vi "Simple TCP - Client.vi"() -> ()   [LabVIEW 2017]
doc: "Demonstrates how to open a connection to an TCP server, read the data being sent, and display the data on a chart. This VI is designed to stop if the TCP connection is terminated."
panel:
  in  "Send":bool
  in  "TCP Send":string
  out "TCP Received":string
  in  "Stop":bool
  # "Overview: Demonstrates the use of the TCP functions to connect to a TCP server VI and receive data.\nInstructions:\n1. Ensure CSM Call and Monitor TCP Traffic.vi or  CSM TCP Server SubModule(Beside Loop Support).vi is already running.\n2. Run the VI.\n3. Click Stop to stop the VI. Note that if you stop the server VI, this VI will stop automatically."
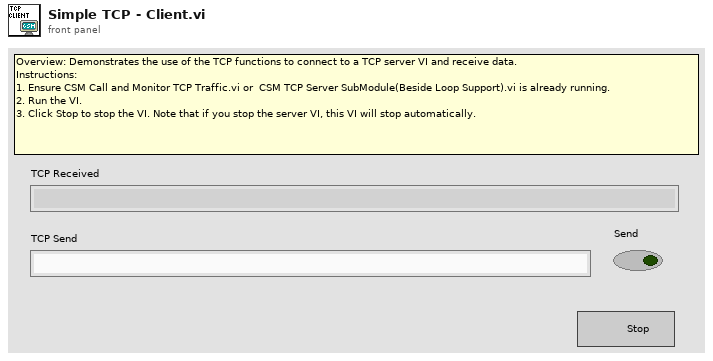
[diagram p1: front panel]
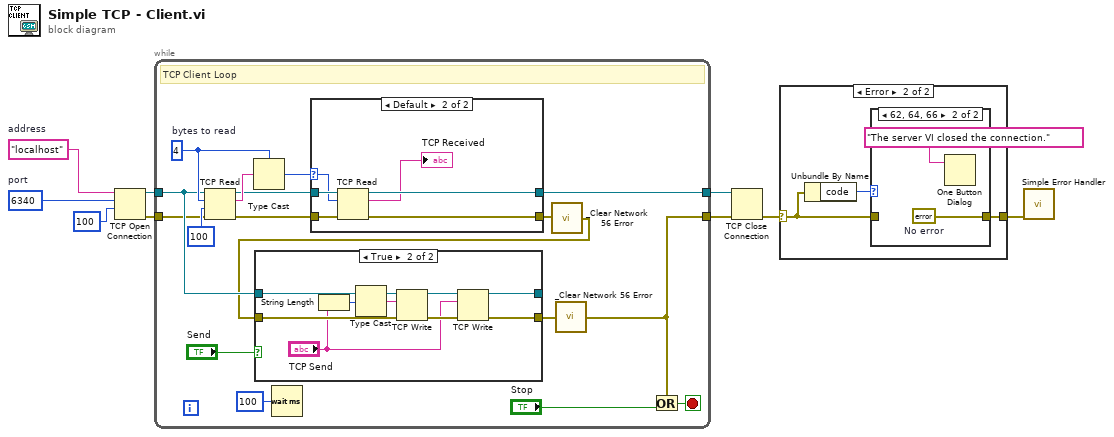
[diagram p0: block diagram]
diagram:
  w4 = u16 6340  # port
  w5 = "localhost"  # address
  n1 = TCP Open Connection(address=w5, remote port or service name=w4, timeout ms (60000)=100 ("timeout ms (25000)")) -> (connection ID=w9:refnum<k5>, error out=w8:errorcluster)  [unwired: 2 in]
  n2 = while {
    tunnel: w8 -> [w14]
    tunnel: w9 -> [w15]
    tunnel: [w12] -> w2
    tunnel: [w10] -> w3
    stop <- w21 stop-if-true
    w23 = 4  # bytes to read
    # "TCP Client Loop"
    n3 = TCP Read(connection ID=w15, bytes to read=w23, error in (no error)=w14, 9:100 ("timeout ms (25000)")) -> (connection ID out=w25:refnum<k5>, data out=w26:string, error out=w24:errorcluster)  [unwired: 1 in]
    n4 = Type Cast(type=w23, x=w26) -> (*(type *) &x=w19:i32)
    n5 = Wait (ms)(milliseconds to wait=u32 100) -> ()  [unwired: 1 out]
    n6 = case shown="Default" w19 {
      selector: w19 -> [_ w41]
      tunnel: w25 -> [w39 w45]
      tunnel: w24 -> [w38 w44]
      tunnel: [w39 w43] -> w12
      tunnel: [w38 w42] -> w13
      frame ..0 {
        # "The server has not written any data"
      }
      frame Default {
        n7 = TCP Read(connection ID=w45, bytes to read=w41, error in (no error)=w44) -> (connection ID out=w43:refnum<k5>, data out=→"TCP Received":string, error out=w42:errorcluster)  [unwired: 2 in]
      }
    }
    n8 = call "_Clear Network 56 Error.vi"("error in (no error)"=w13) -> ("error out"=w11:errorcluster)  [unwired: 4 in]
    n9 = case shown="True" "Send" {
      tunnel: w15 -> [w28 w37]
      tunnel: w11 -> [w27 w34]
      tunnel: [w27 w33] -> w16
      tunnel: [w28 w32] -> _
      frame False {
      }
      frame True {
        n10 = String Length(string="TCP Send") -> (length=w31:i32)
        n11 = Type Cast(x=w31) -> (*(type *) &x=w29:string)  [unwired: 1 in]
        n12 = TCP Write(connection ID=w37, data in=w29, error in (no error)=w34) -> (connection ID out=w36:refnum<k5>, error out=w35:errorcluster)  [unwired: 1 in, 1 out]
        n13 = TCP Write(connection ID=w36, data in="TCP Send", error in (no error)=w35) -> (connection ID out=w32:refnum<k5>, error out=w33:errorcluster)  [unwired: 1 in, 1 out]
      }
    }
    n14 = call "_Clear Network 56 Error.vi"("error in (no error)"=w16) -> ("error out"=w10:errorcluster)  [unwired: 4 in]
    n15 = Or(x=w10, y="Stop") -> (x .or. y?=w21:bool)
  }
  n16 = TCP Close Connection(connection ID=w2, error in (no error)=w3) -> (error out=w7:errorcluster)  [unwired: 1 in, 1 out]
  n17 = case shown="Error" w7 {
    selector: w7 -> [w46 w48]
    tunnel: [w46 w47] -> w6
    frame No Error {
    }
    frame Error {
      n18 = Unbundle By Name(w48) -> ("code"=w49:i32)
      n19 = case shown="62, 64, 66" w49 {
        tunnel: w48 -> [w50 _]
        tunnel: [w50 w52] -> w47
        frame Default {
        }
        frame 62, 64, 66 {
          w52 = errorcluster {"status"=FALSE, "code"=0, "source"=""}  # No error
          n20 = One Button Dialog(message="The server VI closed the connection." ("Server Closed")) -> ()  [unwired: 1 in, 1 out]
        }
      }
    }
  }
  n21 = call <vilib>:"Simple Error Handler.vi"("error in (no error)"=w6) -> ()  [unwired: 4 in, 5 out]
